vi "Get LLM URL.vi"(11 "OpenAI API URL":string="http://localhost:1234/v1" caption="OpenAI API URL (e.g. OpenRouter, LM Studio)") -> (3 "OpenAI API URL":string)   [LabVIEW 2023, in "LabVIEW AI Base.lvlib"]
uses:
  AI Base Globals.vi
  LabVIEW AI Base.lvlib
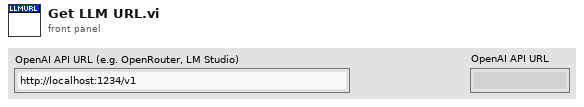
[diagram p1: front panel]
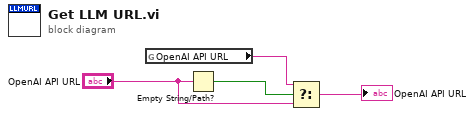
[diagram p0: block diagram]
diagram:
  n1 = global read "AI Base Globals.vi" "OpenAI API URL"() -> (w4:string)
  n2 = Empty String/Path?(string/path="OpenAI API URL") -> (empty?=w3:bool)
  n3 = Select(t=w4, s=w3, f="OpenAI API URL") -> (s? t:f=→"OpenAI API URL":string)
